vi "Create Sheet.vi"(7 "Sheet Name (Sheet1)":string="Sheet1", 8 "error in (no error)":errorcluster, 11 "IWorkbook Reference":refnum<k24>) -> (0 "error out":errorcluster, 2 "Sheet Reference":refnum<k24>, 3 "IWorkbook Reference out":refnum<k24>)   [LabVIEW 2014]
uses:
  C:/Users/LENOVO/Desktop/CodeSpace GUI/LVExcel/Resources/net40/NPOI.dll
  Resources/net40/NPOI.dll
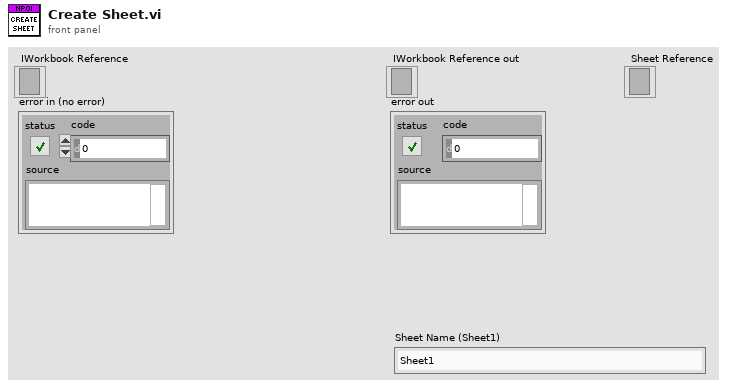
[diagram p1: front panel]
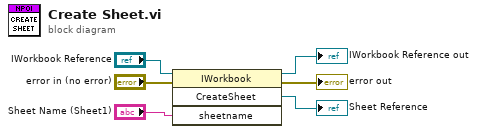
[diagram p0: block diagram]
diagram:
  n1 = invoke class="IWorkbook" method="CreateSheet"(reference="IWorkbook Reference", error in="error in (no error)", "sheetname"="Sheet Name (Sheet1)") -> (reference out=→"IWorkbook Reference out":refnum<k24>, error out=→"error out":errorcluster, "CreateSheet"=→"Sheet Reference":refnum<k24>)  [unwired: 1 in, 1 out]
